vi "Main.vi"() -> ()   [LabVIEW 2014]
doc: "This sample project is built upon the standard state machine template and shows how you could create an application that acquires, analyzes, and presents data. It includes functionality for presenting configuration dialogs, preserving settings between executions, loading and saving data, as well as exporting graph images and text files.\n\nIt is most appropriate for data that is acquired instantly as it does not allow for screen updates mid acquisition nor does it allow for continuous streaming to disk."
uses:
  controls/DAQSettings.ctl
  controls/TriggerMode.ctl
  controls/AspicSettings.ctl
  controls/AspicMode.ctl
  controls/Timeslice.ctl
  controls/SystemSet.ctl
  controls/State.ctl
  controls/Data.ctl
  controls/UI References.ctl
  controls/Graph Data.ctl
  <vilib>/Utility/miscctls.llb/LVAnnotationListTypeDef.ctl
  <vilib>/Utility/miscctls.llb/LVCursorListTypeDef.ctl
  controls/User Specified Data.ctl
  controls/HW Configuration.ctl
  controls/Simulated Signal Type.ctl
  controls/Analysis Configuration.ctl
  controls/New Data Behavior.ctl
  controls/Network.ctl
  controls/CommSelect.ctl
panel:
  out "size(s)":i32[](array[numeric])
  in  "Single channel":bool
  in  "Enum":T1(ring)
  out "System Set":T2
  in  "SystemSet":bool
  in  "DAQSettings":bool
  in  "Timeslice":bool
  in  "Path settings":bool
  in  "Network Settings":bool
  in  "ASPIC Settings":bool
  in  "Snapshot":bool
  in  "Analyze":bool
  in  "Clear":bool
  in  "Exit":bool
  in  "Acquire":bool
  in  "Export":bool
  in  "Save Data":bool
  in  "Load Data":bool
  out "Graph 12":waveform(dbl)[](graph)
  out "Graph 11":waveform(dbl)[](graph)
  out "Graph 10":waveform(dbl)[](graph)
  out "Graph 9":waveform(dbl)[](graph)
  out "Graph 8":waveform(dbl)[](graph)
  out "Graph 7":waveform(dbl)[](graph)
  out "Graph 6":waveform(dbl)[](graph)
  out "Graph 5":waveform(dbl)[](graph)
  out "Graph 2":waveform(dbl)[](graph)
  out "timeslice":T3
  out "Aspic Seeting":T4 {"RC" format="%b"; "Gain" format="%b"}
  out "DAQ Settings":T6
  out "Graph":waveform(dbl)[](graph)
  out "Status Bar":string
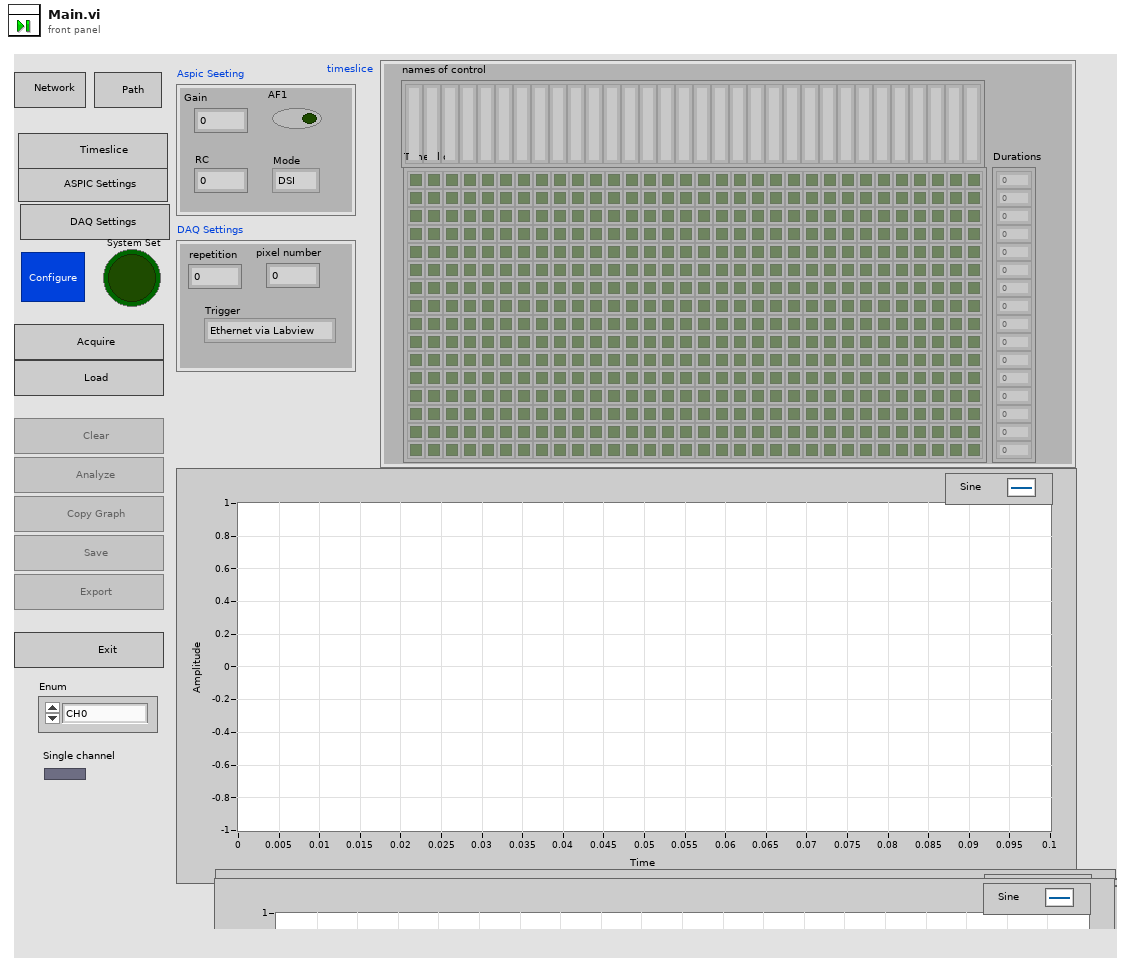
[diagram p1: front panel]
types:
  T1 = enum16{"CH0", "CH1", "CH2", "CH3", "CH4", "CH5", "CH6", "CH7", "All"}
  T2 = typedef "SystemSet.ctl" = bool
  T3 = typedef "Timeslice.ctl" = cluster{"Time slice":bool[][], "Durations":dbl[], "names of control":string[]}
  T4 = typedef "AspicSettings.ctl" = cluster{"Gain":u8, "RC":u8, "aspic1Data":u32[], "aspic2Data":u32[], "AF1":bool, "Mode":T5}
  T5 = typedef "AspicMode.ctl" = enum16{"DSI", "TM"}
  T6 = typedef "DAQSettings.ctl" = cluster{"pixel number":u32, "repetition":u32, "Trigger":T7}
  T7 = typedef "TriggerMode.ctl" = enum16{"Ethernet via Labview", "SMA (1.8V)"}
  T8 = typedef "Data.ctl" = cluster{"UI References":T9, "Graph Data":T10, "User Specified":T13, "Aspic Seeting":T4, "Network":T18, "timeslice":T3, "Acquisition Settings":T6, "CommSelect":T19, "System Set":T2}
  T9 = typedef "UI References.ctl" = cluster{"Exit Ref":refnum<vi>, "Save Ref":refnum<vi>, "Open Ref":refnum<vi>, "Export Ref":refnum<vi>, "Acquire Ref":refnum<vi>, "Configure Ref":refnum<vi>, "Graph Ref":refnum<vi>, "Clear Ref":refnum<vi>, "Analyze Ref":refnum<vi>, "Status Ref":refnum<vi>, "Snapshot Ref":refnum<vi>, "Network Ref":refnum<vi>, "Timeslice Ref":refnum<vi>, "DAQSetting Ref":refnum<vi>, "SystemSet":refnum<vi>}
  T10 = typedef "Graph Data.ctl" = cluster{"Data":waveform(dbl)[], "Annotation List":T11, "Cursor List":T12, "Analysis Data":waveform(dbl)[]}
  T11 = typedef "LVAnnotationListTypeDef.ctl" = cluster{"Name":string, "Color":u32, "Style":u8, "Point Style":u8, "Name Visible":bool, "Allow Drag":bool, "Annotation Mode":u32, "Plot":i32, "Index":i32, "Position":cluster{"X":dbl, "Y":dbl}, "X Scale":u32, "Y Scale":u32, "Show Arrow":bool, "Lock Name":bool, "Plot Area":i32, "Label Offset":cluster{"X":dbl, "Y":dbl}}[]
  T12 = typedef "LVCursorListTypeDef.ctl" = cluster{"Name":string, "Color":u32, "Style":u8, "Point Style":u8, "Name Visible":bool, "Allow Drag":bool, "Cursor Mode":u32, "Plot":i32, "Index":i32, "Position":cluster{"X":dbl, "Y":dbl}, "X Scale":u32, "Y Scale":u32, "Watch Plots":i32[], "Watch All Plots":bool, "Plot Area":i32, "Label Offset":cluster{"X":dbl, "Y":dbl}}[]
  T13 = typedef "User Specified Data.ctl" = cluster{"Hardware Configuration":T14, "Analysis Configuration":T16, "New Data Behavior":T17}
  T14 = typedef "HW Configuration.ctl" = cluster{"HW Refnum <Replace Me>":string, "Signal Type <Replace Me>":T15}
  T15 = typedef "Simulated Signal Type.ctl" = enum16{"Sine Wave", "Square Wave"}
  T16 = typedef "Analysis Configuration.ctl" = cluster{"Statistics":bool}
  T17 = typedef "New Data Behavior.ctl" = enum16{"Replace", "Overlay", "Append"}
  T18 = typedef "Network.ctl" = cluster{"invert_send":bool, "Number of datagrams to read":u32, "max bytes/read":i32, "Timeout":i32, "host":string, "Port Receive":u16}
  T19 = typedef "CommSelect.ctl" = enum16{"startTSL", "writeCABAC", "readCABAC", "resetCABAC", "emissionTest", "regRead", "executeASPIC", "resetASPIC", "resetFifo18ASPIC", "resetFifo16ASPIC", "LabviewDamicStart"}
  T20 = typedef "State.ctl" = enum16{"Initialize", "Wait for Event", "Update UI", "Network", "Configure", "DAQSettings", "Timeslice", "Set Sytem", "Acquire", "Load Data", "Save Data", "Clear Data", "Export Data", "Analyze", "Copy Graph", "Exit"}
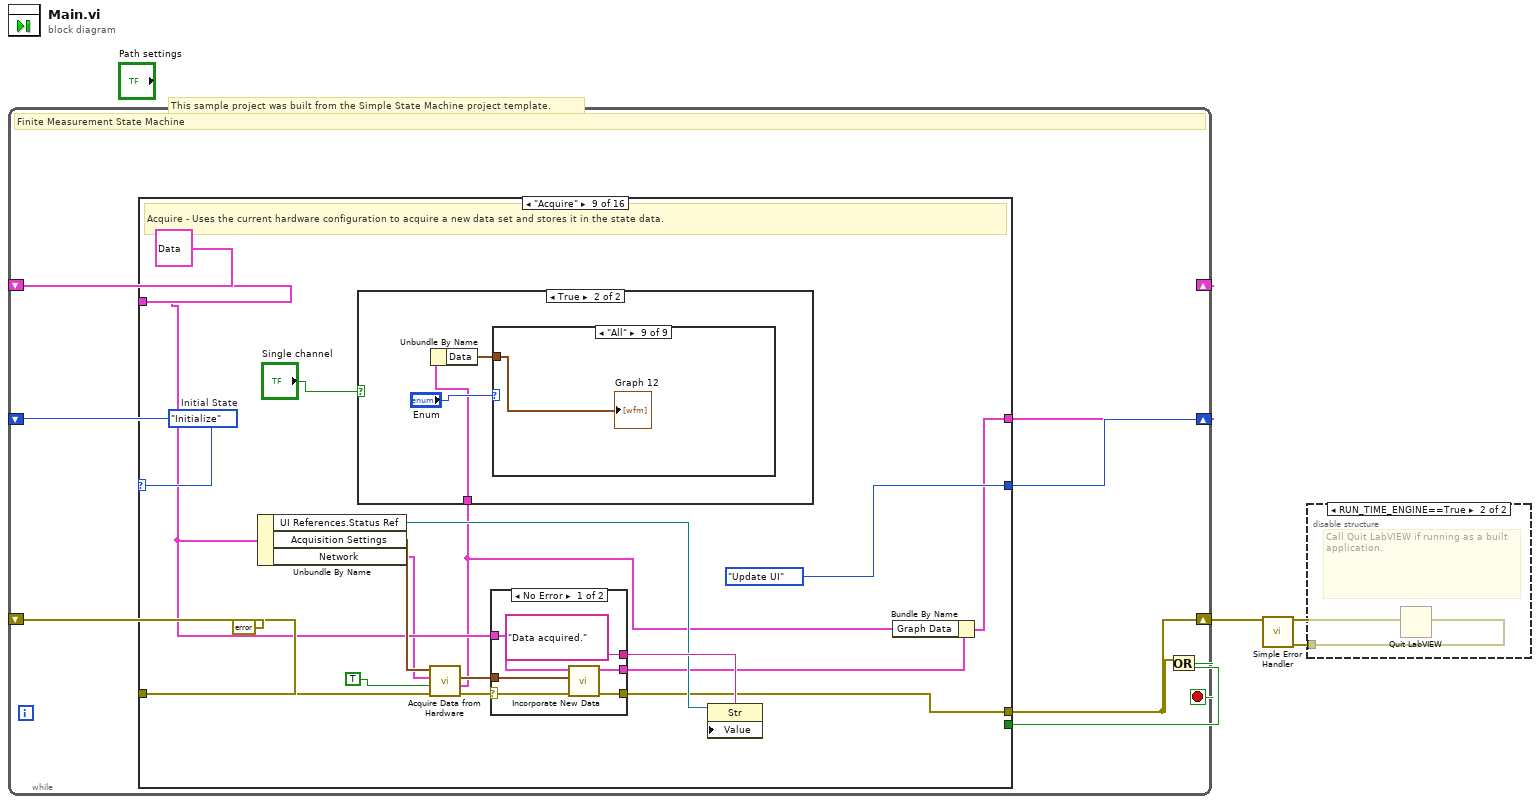
[diagram p0: block diagram]
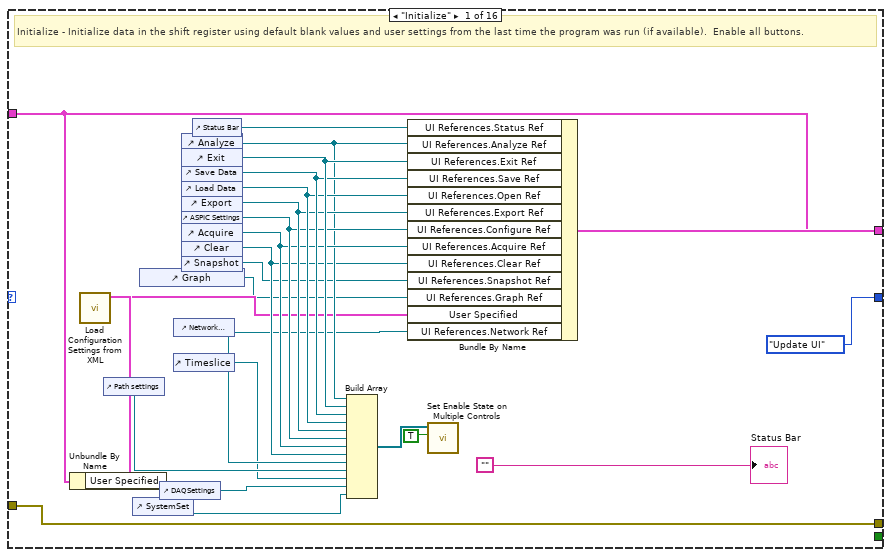
[diagram p3: hidden frame]
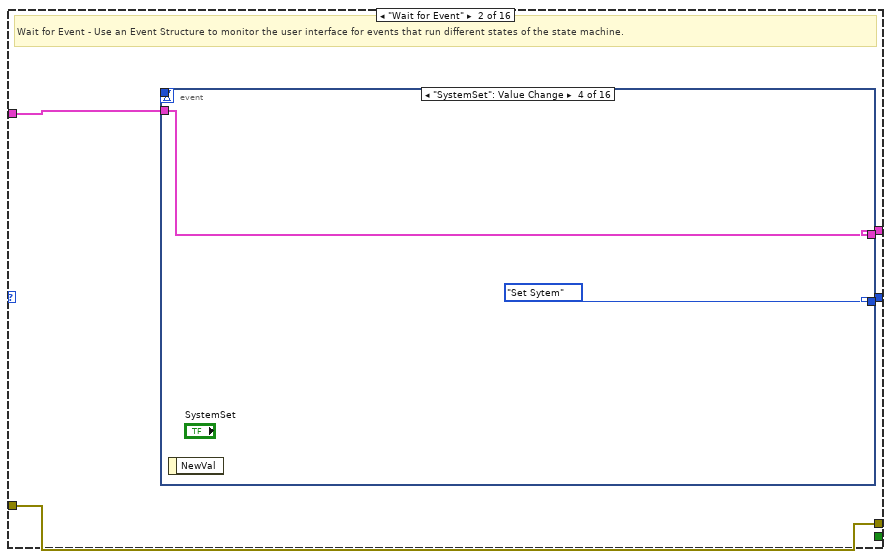
[diagram p4: hidden frame]
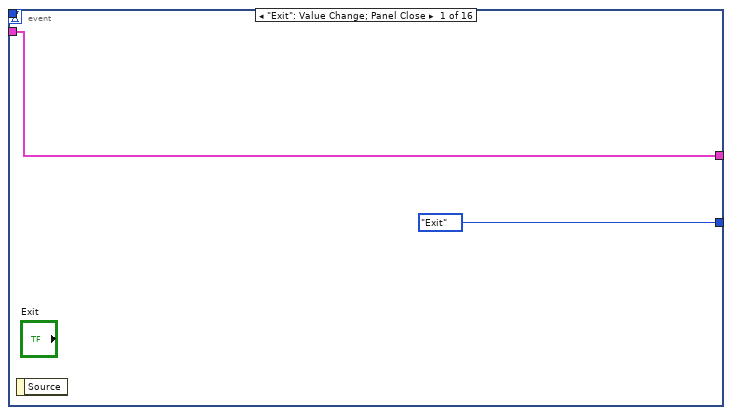
[diagram p5: hidden frame]
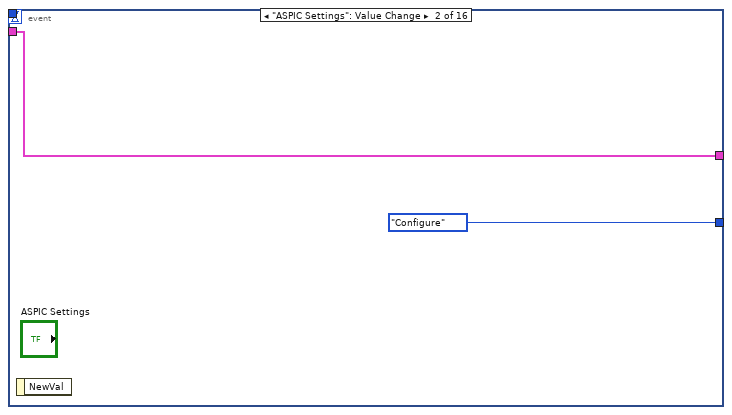
[diagram p6: hidden frame]
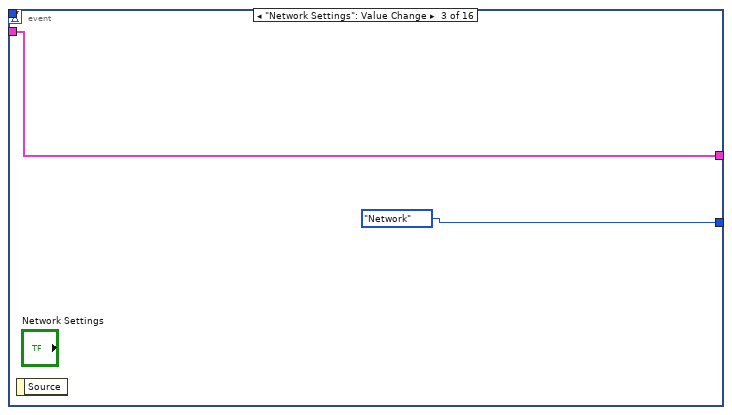
[diagram p7: hidden frame]
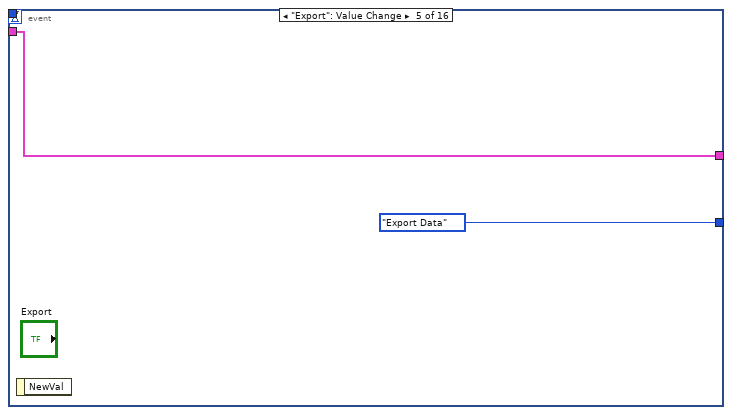
[diagram p8: hidden frame]
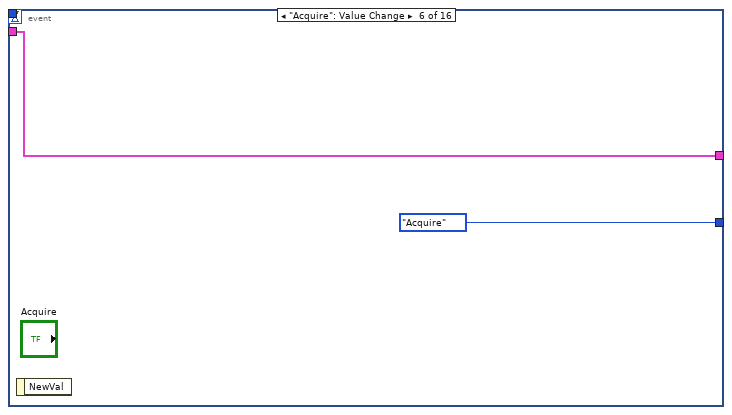
[diagram p9: hidden frame]
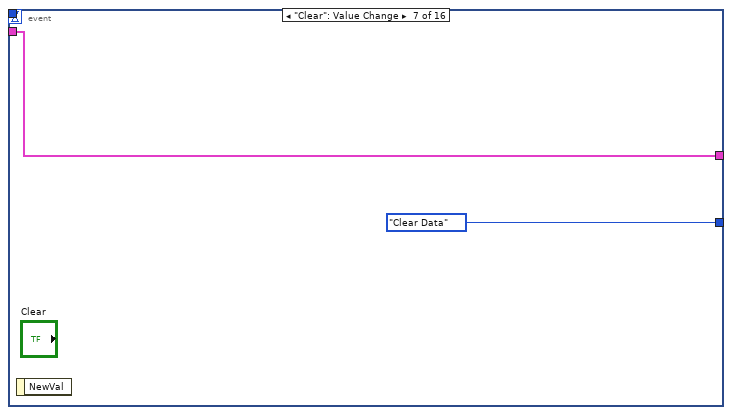
[diagram p10: hidden frame]
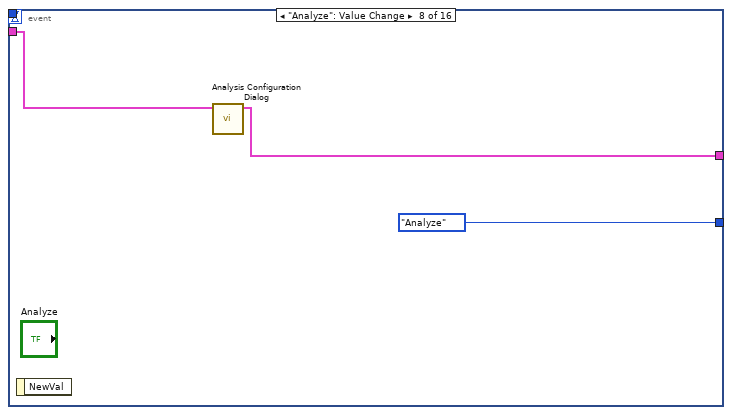
[diagram p11: hidden frame]
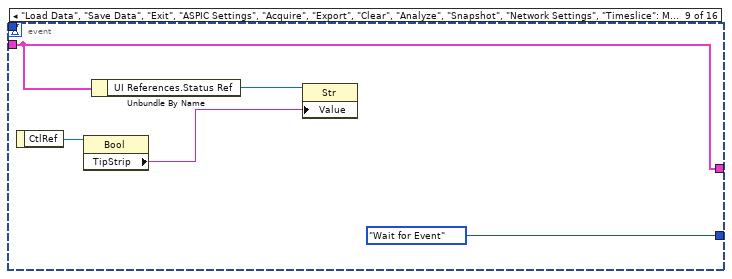
[diagram p12: hidden frame]
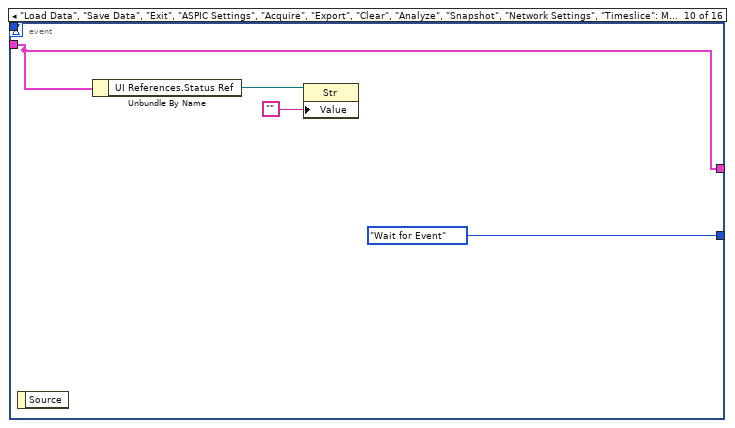
[diagram p13: hidden frame]
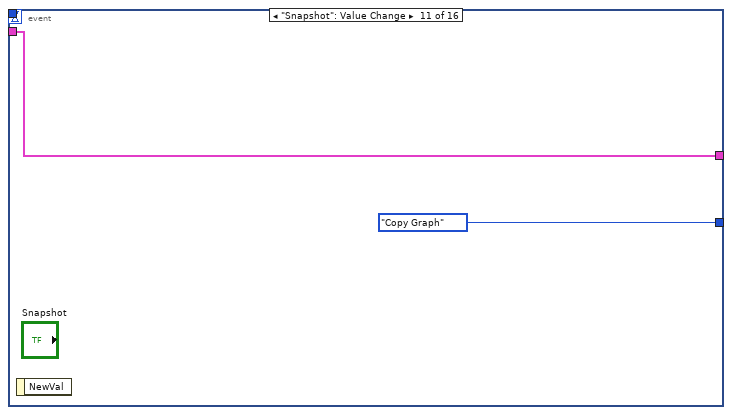
[diagram p14: hidden frame]
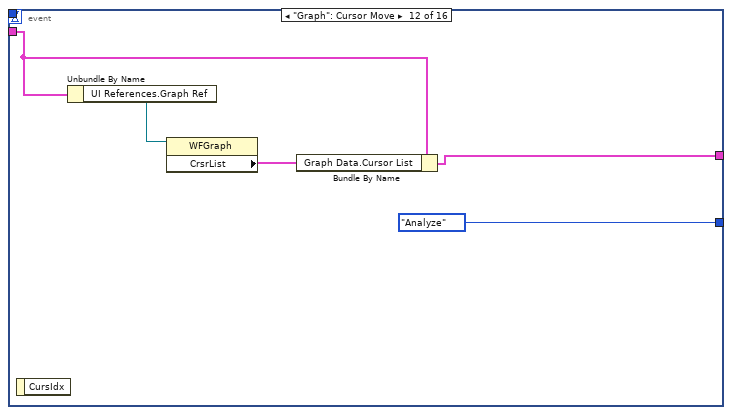
[diagram p15: hidden frame]
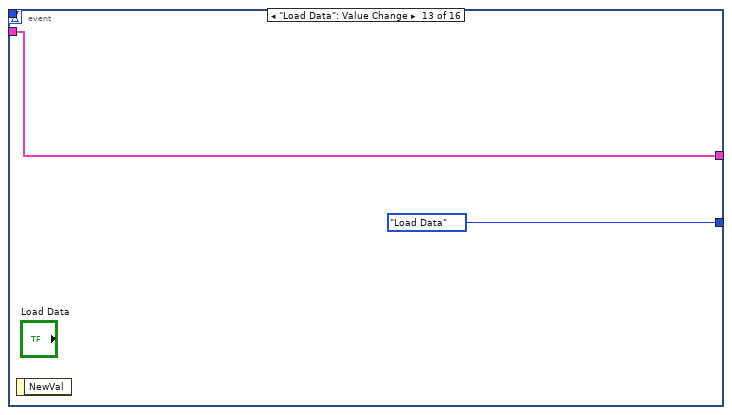
[diagram p16: hidden frame]
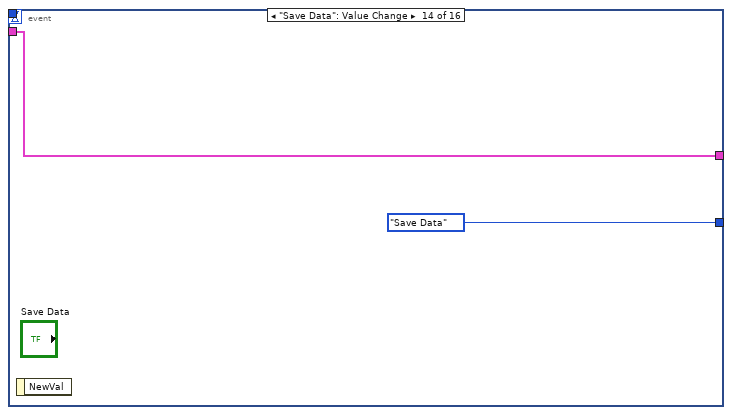
[diagram p17: hidden frame]
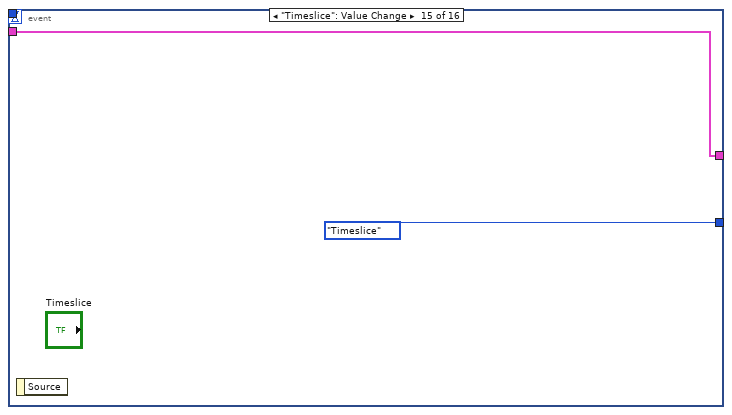
[diagram p18: hidden frame]
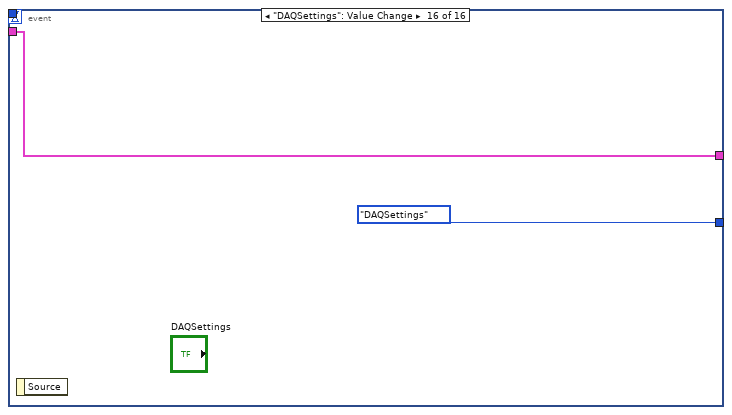
[diagram p19: hidden frame]
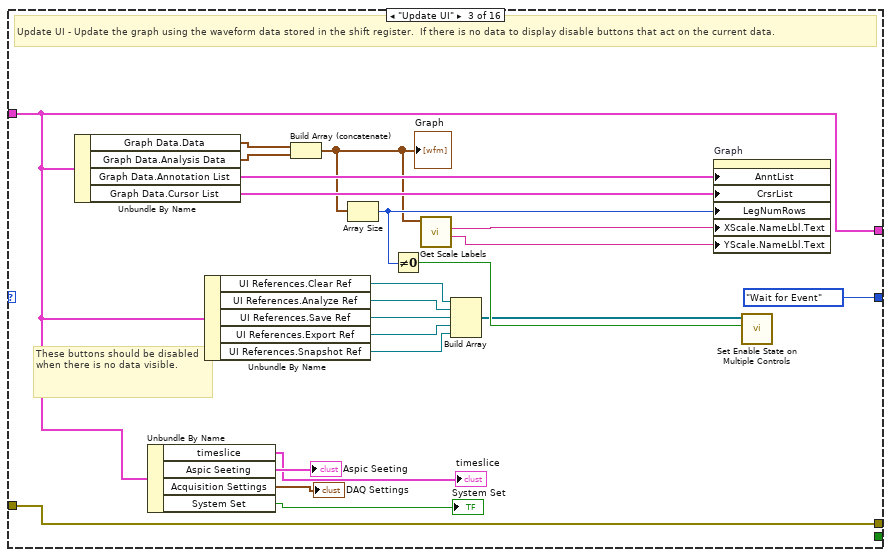
[diagram p20: hidden frame]
diagram:
  w5 = State."Initialize"  # Initial State
  # "This sample project was built from the Simple State Machine project template."
  n1 = while {
    shift-right: [w12] -> _
    shift-left: w5 -> [w13]
    shift-right: [w6] -> w3
    shift-left: errorcluster {"status"=FALSE, "code"=0, "source"=""} ("error constant") -> [w7]
    shift-right: [w8] -> _
    shift-left: T8 {"UI References"={"Exit Ref"=refnum, "Save Ref"=refnum, "Open Ref"=refnum, "Export Ref"=refnum, "Acquire Ref"=refnum, "Configure Ref"=refnum, "Graph Ref"=refnum, "Clear Ref"=refnum, "Analyze Ref"=refnum, "Status Ref"=refnum, "Snapshot Ref"=refnum, "Network Ref"=refnum, "Timeslice Ref"=refnum, "DAQSetting Ref"=refnum, "SystemSet"=refnum}, "Graph Data"={"Data"=[], "Annotation List"=[], "Cursor List"=[], "Analysis Data"=[]}, "User Specified"={"Hardware Configuration"={"HW Refnum <Replace Me>"="", "Signal Type <Replace Me>"=enum."Sine Wave"}, "Analysis Configuration"={"Statistics"=TRUE}, "New Data Behavior"=enum."Replace"}, "Aspic Seeting"={"Gain"=0, "RC"=0, "aspic1Data"=[], "aspic2Data"=[], "AF1"=FALSE, "Mode"=enum."TM"}, "Network"={"invert_send"=TRUE, "Number of datagrams to read"=5000, "max bytes/read"=2500, "Timeout"=4000, "host"="192.168.1.18", "Port Receive"=5678}, "timeslice"={"Time slice"=[], "Durations"=[], "names of control"=[]}, "Acquisition Settings"={"pixel number"=0, "repetition"=0, "Trigger"=enum."Ethernet via Labview"}, "CommSelect"=enum."resetFifo18ASPIC", "System Set"=FALSE} ("Data") -> [w9]
    stop <- w10 stop-if-true
    # "Finite Measurement State Machine"
    n2 = case shown="\"Acquire\"" w13 {
      tunnel: [State."Update UI" ("Next State") w42 State."Wait for Event" ("(Value Not Used)") w107 State."Update UI" ("Next State if true") State."Update UI" ("Next State if true") w143 State."Update UI" ("States") State."Update UI" ("Next State") State."Update UI" ("(Value Not Used)") State."Wait for Event" ("(Value Not Used)") State."Wait for Event" ("(Value Not Used)") State."Update UI" ("(Value Not Used)") State."Update UI" ("(Value Not Used)") State."Wait for Event" ("(Value Not Used)") w287] -> w12
      tunnel: [_ _ _ _ _ _ _ _ _ _ _ _ _ _ _ w286] -> w11
      tunnel: w9 -> [w18 w41 w89 w113 w125 w132 w141 w157 w185 w226 w243 w256 w269 w273 w278 w282]
      tunnel: [w19 w40 w89 w112 w117 w126 w135 w153 w177 w225 w243 w256 w268 w273 w278 w282] -> w8
      tunnel: w7 -> [w17 w39 w90 w109 w124 w131 w147 w155 w184 w223 w242 w255 w267 w272 w277 w281]
      tunnel: [w17 w39 w90 w108 w121 w130 w147 w148 w183 w222 w241 w254 w267 w272 w276 w280] -> w6
      frame "Initialize" {
        # "Initialize - Initialize data in the shift register using default blank values and user settings from the last time the program was run (if available).  Enable all buttons."
        n3 = Unbundle By Name(w18) -> ("User Specified"=w30:T13)
        n4 = call "Load Configuration Settings from XML.vi"("User Configuration in"=w30) -> ("User Configuration out"=w25:T13)  [unwired: 9 in, 1 out]
        n5 = control-ref of="Path settings"() -> (w21:refnum<vi>)
        n6 = control-ref of="SystemSet"() -> (w14:refnum<vi>)
        n7 = control-ref of="Graph"() -> (w22:refnum<vi>)
        n8 = control-ref of="DAQSettings"() -> (w15:refnum<vi>)
        n9 = control-ref of="Network Settings"() -> (w20:refnum<vi>)
        n10 = control-ref of="Timeslice"() -> (w16:refnum<vi>)
        n11 = control-ref of="Analyze"() -> (w29:refnum<vi>)
        n12 = control-ref of="Exit"() -> (w37:refnum<vi>)
        n13 = control-ref of="Save Data"() -> (w36:refnum<vi>)
        n14 = control-ref of="Load Data"() -> (w35:refnum<vi>)
        n15 = control-ref of="Export"() -> (w34:refnum<vi>)
        n16 = control-ref of="ASPIC Settings"() -> (w33:refnum<vi>)
        n17 = control-ref of="Acquire"() -> (w32:refnum<vi>)
        n18 = control-ref of="Clear"() -> (w27:refnum<vi>)
        n19 = control-ref of="Snapshot"() -> (w23:refnum<vi>)
        n20 = control-ref of="Status Bar"() -> (w28:refnum<vi>)
        n21 = Build Array(w29, w37, w36, w35, w34, w33, w32, w27, w20, w21, w16, w15, w14) -> (w31:refnum<vi>[])
        n22 = Bundle By Name(cluster=w18, "UI References.Status Ref"=w28, "UI References.Analyze Ref"=w29, "UI References.Exit Ref"=w37, "UI References.Save Ref"=w36, "UI References.Open Ref"=w35, "UI References.Export Ref"=w34, "UI References.Configure Ref"=w33, "UI References.Acquire Ref"=w32, "UI References.Clear Ref"=w27, "UI References.Snapshot Ref"=w23, "UI References.Graph Ref"=w22, "User Specified"=w25, "UI References.Network Ref"=w20) -> (w19:T8)
        n23 = call "Set Enable State on Multiple Controls.vi"("Enable?"=TRUE, "Controls"=w31) -> ()  [unwired: 10 in]
        "Status Bar" <- "" ("Status Bar")
      }
      frame "Wait for Event" {
        # "Wait for Event - Use an Event Structure to monitor the user interface for events that run different states of the state machine."
        n24 = event shown="[3] \"SystemSet\": Value Change" {
          selector: _ -> [_ _ _ _ _ _ _ _ _ _ _ _ _ _ _ _]
          dyn-events: _ -> [_ _ _ _ _ _ _ _ _ _ _ _ _ _ _ _]
          timeout: _ -> [_ w46 _ _ _ _ _ _ _ _ _ _ _ _ _ _]
          tunnel: [State."Exit" ("Next State") State."Configure" ("Next State") State."Network" ("States") State."Set Sytem" ("States") State."Export Data" ("Next State") State."Acquire" ("Next State") State."Clear Data" ("Next State") State."Analyze" ("Next State") State."Wait for Event" ("Next State") State."Wait for Event" ("Next State") State."Copy Graph" ("Next State") State."Analyze" ("Next State") State."Load Data" ("Next State") State."Save Data" ("Next State") State."Timeslice" ("States") State."DAQSettings" ("States")] -> w42
          tunnel: [_ w46 _ _ _ _ _ _ _ _ _ _ _ _ _ _] -> _
          tunnel: w41 -> [w43 w45 w49 w51 w52 w54 w56 w59 w61 w66 w70 w73 w77 w79 w82 w84]
          tunnel: [w43 w45 w49 w51 w52 w54 w56 w58 w61 w66 w70 w72 w77 w79 w82 w84] -> w40
          event "Exit": Value Change; Panel Close {
            n25 = event-data() -> ()  [unwired: 1 in, 1 out]
          }
          event "ASPIC Settings": Value Change {
            n26 = event-data() -> ()  [unwired: 1 in, 1 out]
          }
          event "Network Settings": Value Change {
            n27 = event-data() -> ()  [unwired: 1 in, 1 out]
          }
          event "SystemSet": Value Change {
            n28 = event-data() -> ()  [unwired: 1 in, 1 out]
          }
          event "Export": Value Change {
            n29 = event-data() -> ()  [unwired: 1 in, 1 out]
          }
          event "Acquire": Value Change {
            n30 = event-data() -> ()  [unwired: 1 in, 1 out]
          }
          event "Clear": Value Change {
            n31 = event-data() -> ()  [unwired: 1 in, 1 out]
          }
          event "Analyze": Value Change {
            n32 = event-data() -> ()  [unwired: 1 in, 1 out]
            n33 = call "Analysis Configuration Dialog.vi"("Data In"=w59) -> ("Data out"=w58:T8)  [unwired: 10 in]
          }
          event "Load Data", "Save Data", "Exit", "ASPIC Settings", "Acquire", "Export", "Clear", "Analyze", "Snapshot", "Network Settings", "Timeslice": Mouse Enter {
            n34 = event-data() -> ("CtlRef"=w65:refnum<vi>)  [unwired: 1 in]
            n35 = property class="Bool"(reference=w65) -> ("TipStrip"=w63:string)  [unwired: 1 in, 2 out]
            n36 = Unbundle By Name(w61) -> ("UI References.Status Ref"=w64:refnum<vi>)
            n37 = property class="Str"(reference=w64, "Value"=w63) -> ()  [unwired: 1 in, 2 out]
          }
          event "Load Data", "Save Data", "Exit", "ASPIC Settings", "Acquire", "Export", "Clear", "Analyze", "Snapshot", "Network Settings", "Timeslice": Mouse Leave {
            n38 = event-data() -> ()  [unwired: 1 in, 1 out]
            n39 = Unbundle By Name(w66) -> ("UI References.Status Ref"=w69:refnum<vi>)
            n40 = property class="Str"(reference=w69, "Value"="") -> ()  [unwired: 1 in, 2 out]
          }
          event "Snapshot": Value Change {
            n41 = event-data() -> ()  [unwired: 1 in, 1 out]
          }
          event "Graph": Cursor Move {
            n42 = event-data() -> ()  [unwired: 1 in, 1 out]
            n43 = Unbundle By Name(w73) -> ("UI References.Graph Ref"=w75:refnum<vi>)
            n44 = property class="WFGraph"(reference=w75) -> ("CrsrList"=w74:T12)  [unwired: 1 in, 2 out]
            n45 = Bundle By Name(cluster=w73, "Graph Data.Cursor List"=w74) -> (w72:T8)
          }
          event "Load Data": Value Change {
            n46 = event-data() -> ()  [unwired: 1 in, 1 out]
          }
          event "Save Data": Value Change {
            n47 = event-data() -> ()  [unwired: 1 in, 1 out]
          }
          event "Timeslice": Value Change {
            n48 = event-data() -> ()  [unwired: 1 in, 1 out]
          }
          event "DAQSettings": Value Change {
            n49 = event-data() -> ()  [unwired: 1 in, 1 out]
          }
        }
      }
      frame "Update UI" {
        # "These buttons should be disabled when there is no data visible."
        # "Update UI - Update the graph using the waveform data stored in the shift register.  If there is no data to display disable buttons that act on the current data."
        n50 = Unbundle By Name(w89) -> ("Graph Data.Data"=w94:waveform(dbl)[], "Graph Data.Analysis Data"=w93:waveform(dbl)[], "Graph Data.Annotation List"=w96:T11, "Graph Data.Cursor List"=w95:T12)
        n51 = Unbundle By Name(w89) -> ("timeslice"=→"timeslice":T3, "Aspic Seeting"=→"Aspic Seeting":T4, "Acquisition Settings"=→"DAQ Settings":T6, "System Set"=→"System Set":T2)
        n52 = Unbundle By Name(w89) -> ("UI References.Clear Ref"=w102:refnum<vi>, "UI References.Analyze Ref"=w101:refnum<vi>, "UI References.Save Ref"=w105:refnum<vi>, "UI References.Export Ref"=w99:refnum<vi>, "UI References.Snapshot Ref"=w100:refnum<vi>)
        n53 = Build Array (concatenate)(w94, w93) -> (w92:waveform(dbl)[])
        "Graph" <- w92
        n54 = Array Size(array=w92) -> (size(s)=w104:i32)
        n55 = Not Equal To 0?(x=w104) -> (x != 0?=w103:bool)
        n56 = call "Get Scale Labels.vi"("Array of Waveforms"=w92) -> ("Y Scale Label Text"=w97:string, "X Scale Label Text"=w98:string)  [unwired: 9 in]
        n57 = Build Array(w102, w101, w105, w99, w100) -> (w91:refnum<vi>[])
        n58 = property on="Graph" class="WFGraph (strict)"("AnntList"=w96, "CrsrList"=w95, "LegNumRows"=w104, "XScale.NameLbl.Text"=w98, "YScale.NameLbl.Text"=w97) -> ()  [unwired: 2 in, 2 out]
        n59 = call "Set Enable State on Multiple Controls.vi"("Enable?"=w103, "Controls"=w91) -> ()  [unwired: 10 in]
      }
      frame "Network" {
        n60 = Unbundle By Name(w113) -> ("Network"=w114:T18)
        n61 = call "NetworkSettingsDialog.vi"("error in (no error)"=w109, "Network In"=w114) -> ("error out"=w108:errorcluster, "UI Refresh Needed?"=w110:bool, "Network Out"=w111:T18)  [unwired: 7 in]
        n62 = Bundle By Name(cluster=w113, "Network"=w111) -> (w112:T8)
        n63 = Select(t=State."Update UI" ("Next State if true"), s=w110, f=State."Wait for Event" ("Next State if false")) -> (s? t:f=w107:T20)
      }
      frame "Configure" {
        # "Configure - Spawns a dialog that allows the user to set any user configurable settings."
        n64 = Unbundle By Name(w125) -> ("Aspic Seeting"=w123:T4)
        n65 = call "AspicSettingsDialog.vi"("error in (no error)"=w124, "Aspic Seeting In"=w123) -> ("error out"=w121:errorcluster, "Aspic Seeting Out"=w122:T4)  [unwired: 5 in, 1 out]
        n66 = Bundle By Name(cluster=w125, "Aspic Seeting"=w122) -> (w118:T8)
        n67 = Bundle By Name(cluster=w118, "System Set"=FALSE) -> (w117:T8)
      }
      frame "DAQSettings" {
        n68 = Unbundle By Name(w132) -> ("Acquisition Settings"=w134:T6)
        n69 = call "DAQSettingsDialog.vi"("error in (no error)"=w131, "Acquisition Settings In"=w134) -> ("error out"=w130:errorcluster, "Acquisition Settings Out"=w133:T6)  [unwired: 7 in, 1 out]
        n70 = Bundle By Name(cluster=w132, "Acquisition Settings"=w133) -> (w127:T8)
        n71 = Bundle By Name(cluster=w127, "System Set"=FALSE) -> (w126:T8)
      }
      frame "Timeslice" {
        n72 = Unbundle By Name(w141) -> ("timeslice"=w142:T3)
        n73 = call "SetTimesliceDialog.vi"("timeslice in"=w142) -> ("timeslice out"=w140:T3)  [unwired: 10 in]
        n74 = Bundle By Name(cluster=w141, "timeslice"=w140) -> (w136:T8)
        n75 = Unbundle By Name(w136) -> ("timeslice.Time slice"=w139:bool[][])
        n76 = Array Size(array=w139) -> (size(s)=→"size(s)":i32[])
        n77 = Select(t=State."Update UI" ("Next State if true"), s=TRUE, f=State."Wait for Event" ("Next State if false")) -> (s? t:f=w143:T20)
        n78 = Bundle By Name(cluster=w136, "System Set"=FALSE) -> (w135:T8)
      }
      frame "Set Sytem" {
        # "reset the FIFO of the FPGA"
        # "ASPIC gain / RC etc"
        n79 = flat-sequence {
          tunnel: w157 -> [w162]
          tunnel: [w160] -> w156
          tunnel: w155 -> [_]
          tunnel: [w159] -> w154
          tunnel: w156 -> [w169]
          tunnel: w154 -> [w168]
          tunnel: [w169] -> w151
          tunnel: [w164] -> w149
          tunnel: w151 -> [w171]
          tunnel: [w171] -> w150
          tunnel: w149 -> [w170]
          tunnel: [w170] -> w148
          tunnel: [w174] -> w153
          tunnel: w150 -> [w176]
          frame #0 {
            n80 = Unbundle By Name(w162) -> ("Aspic Seeting"=w163:T4, "Acquisition Settings"=w158:T6)
            n81 = call "SetASPIC.vi"("Acquisition Settings"=w158, "Aspic Seeting In"=w163) -> ("error out"=w159:errorcluster, "Aspic Seeting Out"=w161:T4)  [unwired: 8 in]
            n82 = Bundle By Name(cluster=w162, "Aspic Seeting"=w161) -> (w160:T8)
          }
          frame #1 {
            n83 = call "programComm.vi"("error in (no error)"=w168, "CommSelect"=CommSelect."resetFifo16ASPIC") -> ("error out"=w165:errorcluster)
            n84 = call "programComm.vi"("error in (no error)"=w165, "CommSelect"=CommSelect."resetFifo18ASPIC") -> ("error out"=w164:errorcluster)
          }
          frame #2 {
            n85 = Unbundle By Name(w171) -> ("timeslice"=w173:T3, "Acquisition Settings"=w172:T6)
            n86 = call "SetTS.vi"("Acquisition Settings"=w172, "timeslice"=w173) -> ()  [unwired: 10 in]
          }
          frame #3 {
            n87 = Bundle By Name(cluster=w176, "System Set"=TRUE) -> (w174:T8)
          }
        }
      }
      frame "Acquire" {
        # "Acquire - Uses the current hardware configuration to acquire a new data set and stores it in the state data."
        n88 = Unbundle By Name(w185) -> ("UI References.Status Ref"=w186:refnum<vi>, "Acquisition Settings"=w190:T6, "Network"=w182:T18)
        n89 = call "Acquire Data from Hardware.vi"("error in (no error)"=w184, "read"=TRUE, "Network"=w182, "Acquisition Settings"=w190) -> ("error out"=w187:errorcluster, "Graph Data 2"=w178:T10, "Graph Data"=w188:waveform(dbl)[])  [unwired: 5 in]
        n90 = case shown="True" "Single channel" {
          tunnel: w178 -> [_ w193]
          frame False {
          }
          frame True {
            n91 = Unbundle By Name(w193) -> ("Data"=w192:waveform(dbl)[])
            n92 = case shown="\"All\"" "Enum" {
              tunnel: w192 -> [w195 w198 w200 w202 w204 w206 w208 w210 w211]
              frame "CH0", Default {
                n93 = Decimate 1D Array(w195) -> (→"Graph 5":waveform(dbl)[])  [unwired: 7 out]
              }
              frame "CH1" {
                n94 = Decimate 1D Array(w198) -> (→"Graph 2":waveform(dbl)[])  [unwired: 7 out]
              }
              frame "CH2" {
                n95 = Decimate 1D Array(w200) -> (→"Graph 6":waveform(dbl)[])  [unwired: 7 out]
              }
              frame "CH3" {
                n96 = Decimate 1D Array(w202) -> (→"Graph 7":waveform(dbl)[])  [unwired: 7 out]
              }
              frame "CH4" {
                n97 = Decimate 1D Array(w204) -> (→"Graph 8":waveform(dbl)[])  [unwired: 7 out]
              }
              frame "CH5" {
                n98 = Decimate 1D Array(w206) -> (→"Graph 9":waveform(dbl)[])  [unwired: 7 out]
              }
              frame "CH6" {
                n99 = Decimate 1D Array(w208) -> (→"Graph 10":waveform(dbl)[])  [unwired: 7 out]
              }
              frame "CH7" {
                n100 = Decimate 1D Array(w210) -> (→"Graph 11":waveform(dbl)[])  [unwired: 7 out]
              }
              frame "All" {
                "Graph 12" <- w211
              }
            }
          }
        }
        n101 = case shown="No Error" w187 {
          selector: w187 -> [w215 w221]
          tunnel: [w217 w219] -> w179
          tunnel: w188 -> [w216 _]
          tunnel: ["Data acquired." ("Data acquired") "Data not acquired." ("Data not acquired")] -> w189
          tunnel: w185 -> [w213 w219]
          tunnel: [w212 w218] -> w183
          frame No Error {
            n102 = call "Incorporate New Data.vi"("error in (no error)"=w215, "New Graph Data"=w216, "Data in"=w213) -> ("error out"=w212:errorcluster, "Data out"=w217:T8)  [unwired: 7 in]
          }
          frame Error {
            n103 = call <vilib>:"Simple Error Handler.vi"("error in (no error)"=w221) -> ("error out"=w218:errorcluster)  [unwired: 4 in, 4 out]
          }
        }
        n104 = property class="Str"(reference=w186, "Value"=w189) -> ()  [unwired: 1 in, 2 out]
        n105 = Bundle By Name(cluster=w179, "Graph Data"=w178) -> (w177:T8)
      }
      frame "Load Data" {
        # "Load Data - Loads data from a TDMS file and incorporates it with the existing data according to the user's preference."
        n106 = call "Load Data.vi"("error in (no error)"=w223) -> ("error out"=w229:errorcluster, "New Graph Data"=w227:waveform(dbl)[])  [unwired: 9 in]
        n107 = case shown="No Error" w229 {
          selector: w229 -> [w234 w240]
          tunnel: [w236 w238] -> w225
          tunnel: w227 -> [w235 _]
          tunnel: ["Data loaded." ("Data loaded") "Data not loaded." ("Data not loaded")] -> w228
          tunnel: w226 -> [w232 w238]
          tunnel: [w231 w237] -> w222
          frame No Error {
            n108 = call "Incorporate New Data.vi"("error in (no error)"=w234, "New Graph Data"=w235, "Data in"=w232) -> ("error out"=w231:errorcluster, "Data out"=w236:T8)  [unwired: 7 in]
          }
          frame Error {
            n109 = call <vilib>:"Simple Error Handler.vi"("error in (no error)"=w240) -> ("error out"=w237:errorcluster)  [unwired: 4 in, 4 out]
          }
        }
        n110 = Unbundle By Name(w225) -> ("UI References.Status Ref"=w224:refnum<vi>)
        n111 = property class="Str"(reference=w224, "Value"=w228) -> ()  [unwired: 1 in, 2 out]
      }
      frame "Save Data" {
        # "Save Data - Saves the existing measurement data to a TDMS file."
        n112 = Unbundle By Name(w243) -> ("UI References.Status Ref"=w244:refnum<vi>, "Graph Data.Data"=w245:waveform(dbl)[])
        n113 = call "Save Data.vi"("error in (no error)"=w242, "Data"=w245) -> ("error out"=w247:errorcluster)  [unwired: 9 in]
        n114 = case shown="Error" w247 {
          selector: w247 -> [w249 w253]
          tunnel: ["Data saved." ("Data saved") "Data not saved." ("Data not saved")] -> w246
          tunnel: [w249 w251] -> w241
          frame No Error {
          }
          frame Error {
            n115 = call <vilib>:"Simple Error Handler.vi"("error in (no error)"=w253) -> ("error out"=w251:errorcluster)  [unwired: 4 in, 4 out]
          }
        }
        n116 = property class="Str"(reference=w244, "Value"=w246) -> ()  [unwired: 1 in, 2 out]
      }
      frame "Export Data" {
        # "Export Data - Exports the currently loaded measurement and analysis data to a text file that can be imported into a spreadsheet or other application."
        n117 = Unbundle By Name(w256) -> ("UI References.Status Ref"=w257:refnum<vi>, "Graph Data"=w258:T10)
        n118 = call "Export Data.vi"("error in (no error)"=w255, "Graph Data"=w258) -> ("error out"=w259:errorcluster)  [unwired: 9 in]
        n119 = case shown="No Error" w259 {
          selector: w259 -> [w262 w266]
          tunnel: ["Data exported." ("Data exported") "Data not exported." ("Data not exported")] -> w260
          tunnel: [w262 w264] -> w254
          frame No Error {
          }
          frame Error {
            n120 = call <vilib>:"Simple Error Handler.vi"("error in (no error)"=w266) -> ("error out"=w264:errorcluster)  [unwired: 4 in, 4 out]
          }
        }
        n121 = property class="Str"(reference=w257, "Value"=w260) -> ()  [unwired: 1 in, 2 out]
      }
      frame "Clear Data" {
        # "Clear Data - Clears the data currently in the graph."
        n122 = Bundle By Name(cluster=w269, "Graph Data"=T10 {"Data"=[], "Annotation List"=[], "Cursor List"=[], "Analysis Data"=[]} ("Graph")) -> (w268:T8)
      }
      frame "Analyze" {
        # "#CodeRecommended - Add your own signal analysis here."
        # "Analyze - Analyzes the measurement data."
        n123 = Unbundle By Name(w273) -> ("Graph Data"=w274:T10)
        n124 = call "Statistical Analysis.vi"("Graph Data In"=w274) -> ()  [unwired: 9 in, 2 out]
      }
      frame "Copy Graph" {
        # "Copy Graph - Places an image of the graph on the clipboard for pasting into reports or emails."
        n125 = call "Copy Graph to Clipboard.vi"("error in (no error)"=w277, "Graph Data"=w278) -> ("error out"=w276:errorcluster)  [unwired: 9 in]
      }
      frame "Exit" {
        w286 = TRUE  # Stop Loop?
        w287 = State."Exit"  # (Value Not Used)
        # "Exit - Saves the user's settings to an XML file and stops execution."
        n126 = Unbundle By Name(w282) -> ("UI References.Status Ref"=w283:refnum<vi>, "User Specified"=w284:T13)
        n127 = call "Save Configuration Settings to XML.vi"("error in (no error)"=w281, "User Configuration"=w284) -> ("error out"=w280:errorcluster)  [unwired: 9 in]
        n128 = property class="Str"(reference=w283, "Value"="Application exit." ("Stopped")) -> ()  [unwired: 1 in, 2 out]
      }
    }
    n129 = Or(x=w6, y=w11) -> (x .or. y?=w10:bool)
  }
  n130 = call <vilib>:"Simple Error Handler.vi"("error in (no error)"=w3) -> ("error out"=w2:errorcluster)  [unwired: 4 in, 4 out]
  n131 = disable-structure shown="RUN_TIME_ENGINE==True" {
    disable-tunnel: w2 -> [_ _]
    frame condition #0 (active) {
    }
    frame condition #1 {
      # "Call Quit LabVIEW if running as a built application."
      n132 = Quit LabVIEW() -> ()  [unwired: 1 in]
    }
  }
